vi "Write Digital Display[].vi"(5 "Digital Display[]":refnum<class "Digital.lvclass">[](array[class]), 9 "WaveformChart in":refnum<class "WaveformChart.lvclass">) -> (3 "WaveformChart out":refnum<class "WaveformChart.lvclass">)   [LabVIEW 2014, in "WaveformChart.lvclass"]
uses:
  WaveformChart.lvclass
  Digital/Digital.lvclass
  WaveformChart.lvclass/WaveformChart.ctl
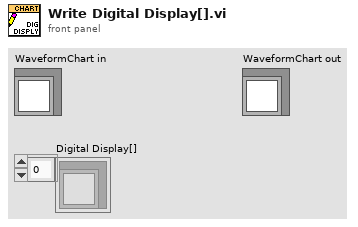
[diagram p1: front panel]
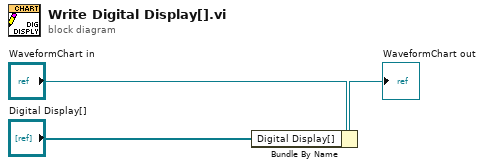
[diagram p0: block diagram]
diagram:
  n1 = Bundle By Name(cluster="WaveformChart in", "Digital Display[]"="Digital Display[]") -> (→"WaveformChart out":refnum<class "WaveformChart.lvclass">)
